vi "Arrange VIWin - Establish Window Bounds.vi"(0 "Window INI tokens":T4, 5 "content rectangle width":i16, 7 "content rectangle height":i16, 11 "error in":errorcluster) -> (4 "window bounds":T1, 15 "error out":errorcluster)   [LabVIEW 2020, in "Arrange VI Window.lvlib"]
uses:
  Arrange VI Window.lvlib
  <vilib>/Utility/miscctls.llb/LVRectTypeDef.ctl
  Arrange VIWin - Min Window Dimensions.ctl
  Arrange VIWin - Window Gaps.ctl
  Arrange VIWin - Rectangle Dimensions.ctl
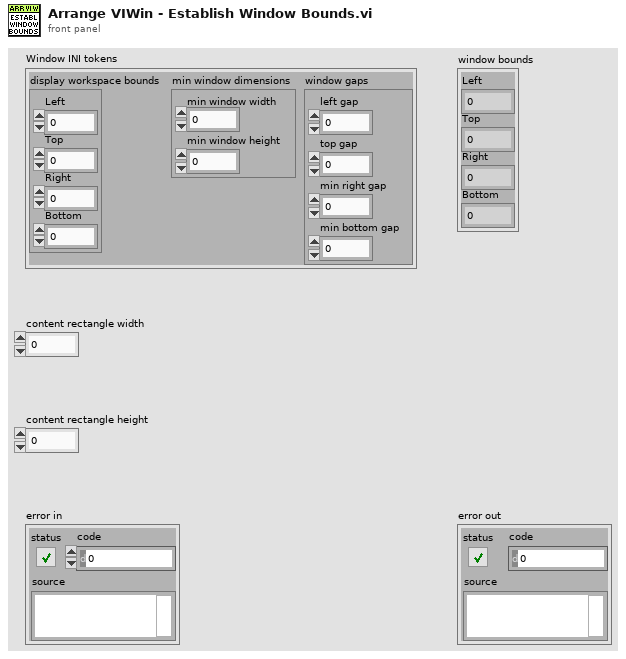
[diagram p1: front panel]
types:
  T1 = typedef "LVRectTypeDef.ctl" = cluster{"Left":i16, "Top":i16, "Right":i16, "Bottom":i16}
  T2 = typedef "Arrange VI Window.lvlib/Arrange VIWin - Min Window Dimensions.ctl" = cluster{"min window width":i16, "min window height":i16}
  T3 = typedef "Arrange VI Window.lvlib/Arrange VIWin - Window Gaps.ctl" = cluster{"left gap":i16, "top gap":i16, "min right gap":i16, "min bottom gap":i16}
  T4 = cluster{"display workspace bounds":T1, "min window dimensions":T2, "window gaps":T3}
  T5 = typedef "Arrange VI Window.lvlib/Arrange VIWin - Rectangle Dimensions.ctl" = cluster{"x":i16, "y":i16}
  T6 = typedef "Arrange VI Window.lvlib/Arrange VIWin - Window Margins.ctl" = cluster{"sum of horizontal margins":i16, "sum of vertical margins":i16}
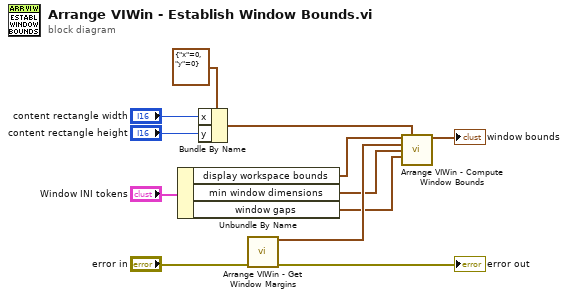
[diagram p0: block diagram]
diagram:
  n1 = Unbundle By Name("Window INI tokens") -> ("display workspace bounds"=w3:T1, "min window dimensions"=w2:T2, "window gaps"=w1:T3)
  n2 = Bundle By Name(cluster=T5 {"x"=0, "y"=0} ("Rectangle Dimensions"), "x"="content rectangle width", "y"="content rectangle height") -> (w8:T5)
  n3 = call "Arrange VIWin - Get Window Margins.vi"("error in"="error in") -> ("window margins"=w7:T6, "error out"=→"error out":errorcluster)  [unwired: 13 in]
  n4 = call "Arrange VIWin - Compute Window Bounds.vi"("display workspace bounds"=w3, "content rectangle"=w8, "window bounds"=w7, "min window dimensions"=w2, "window gaps"=w1) -> ("window bounds"=→"window bounds":T1)  [unwired: 10 in]
